vi "Read Devices Config.vi"() -> (3 "Devices JSON":string)   [LabVIEW 2019, in "SLMP.lvlib"]
uses:
  SLMP.lvlib
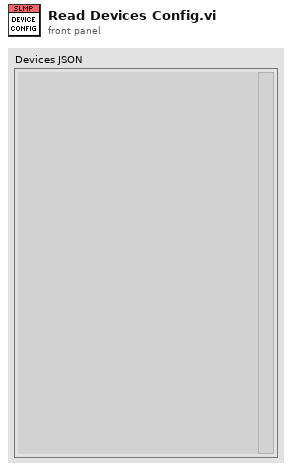
[diagram p1: front panel]
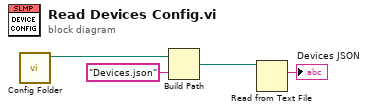
[diagram p0: block diagram]
diagram:
  n1 = call "Config Folder.vi"() -> (".config folder"=w1:path)  [unwired: 11 in]
  n2 = Build Path(base path=w1, name or relative path="Devices.json") -> (appended path=w3:path)
  n3 = Read from Text File(file (use dialog)=w3) -> (text=→"Devices JSON":string)  [unwired: 3 in, 3 out]
